vi "Main_direct.vi"() -> ()   [LabVIEW 2016]
doc: "The myRIO Project template acquires acceleration data from the onboard accelerometer and displays the changes of acceleration values in a waveform chart."
uses:
  <vilib>/FPGAPlugInAG/myRIO-1900/niLvFpga_Open_myRIO-1900.vi
  <vilib>/rvi/interface/common/dynamic/niFpgaDynamicAddResources.vi
  <vilib>/Utility/error.llb/Error Cluster From Error Code.vi
  <vilib>/rvi/errors/niLvFpgaAdjustHostInterfaceError.vi
  <vilib>/FPGAPlugInAG/Dynamic/niLvFpga_Close_Dynamic.vi
  <vilib>/rvi/interface/nirviOpenFPGA/nirviOpenFPGA.xnode
  FPGA Bitfiles/WS2811driver_FPGATarget_FPGAmain_HaK4FqHt+Z8.lvbitx
  <vilib>/rvi/interface/nirviReadWriteControl/nirviReadWriteControl.xnode
  <vilib>/rvi/interface/nirviCloseFPGA/nirviCloseFPGA.xnode
  NiFpgaLv.dll
  <vilib>/rvi/interface/Simulation/niFpgaSimulationCallBeginRW.vi
panel:
  in  "Numeric":u8=1
  out "Numeric Control 2":i32=155
  out "x^2":dbl=0.3694732795078815
  out "Boolean 3":bool=TRUE
  out "Boolean 2":bool
  out "Boolean":bool
  out "Numeric Control":i32=94
  out "appended array":bool[](array[boolean])=[FALSE, FALSE, FALSE, FALSE, FALSE, FALSE, FALSE, FALSE, FALSE, FALSE, FALSE, FALSE, FALSE, FALSE, FALSE, FALSE, FALSE, TRUE, FALSE, TRUE, TRUE, TRUE, TRUE, FALSE]
  in  "Count(mSec)":u32=25
  in  "H0":i32=20
  in  "L1":i32=52
  in  "L0":i32=80
  in  "H1":i32=48
  in  "Enum":enum16{"WS2812", "WS2811", "Debug"}(ring)
  in  "reset ticks)":u32=2000
  in  "number of leds":i32=100
  in  "Stop Button":bool
  out "error out":errorcluster={"status"=FALSE, "code"=-2220, "source"=""}
  # "Overview: The myRIO Project template acquires acceleration data from the onboard accelerometer and displays the changes of acceleration values in a waveform chart.\nInstructions:\n1. Check the myRIO target IP address in the project and make sure the target IP address is correct. \n2. Run this VI."
  # "g"
  # "b"
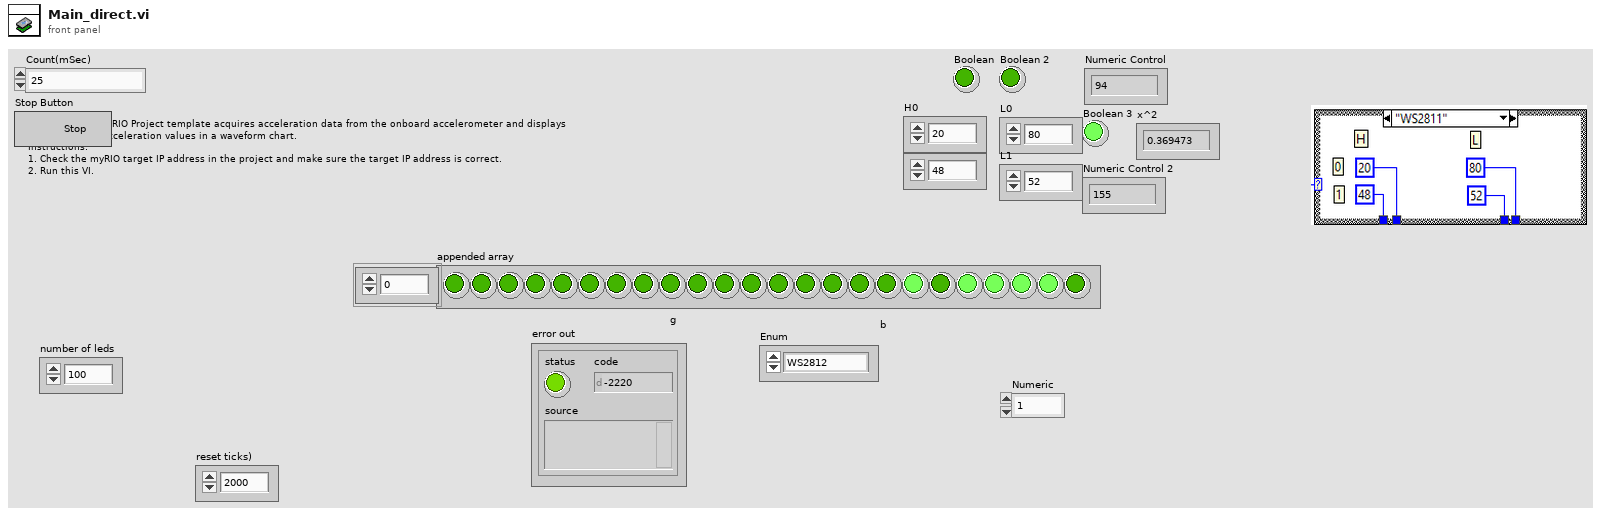
[diagram p1: front panel]
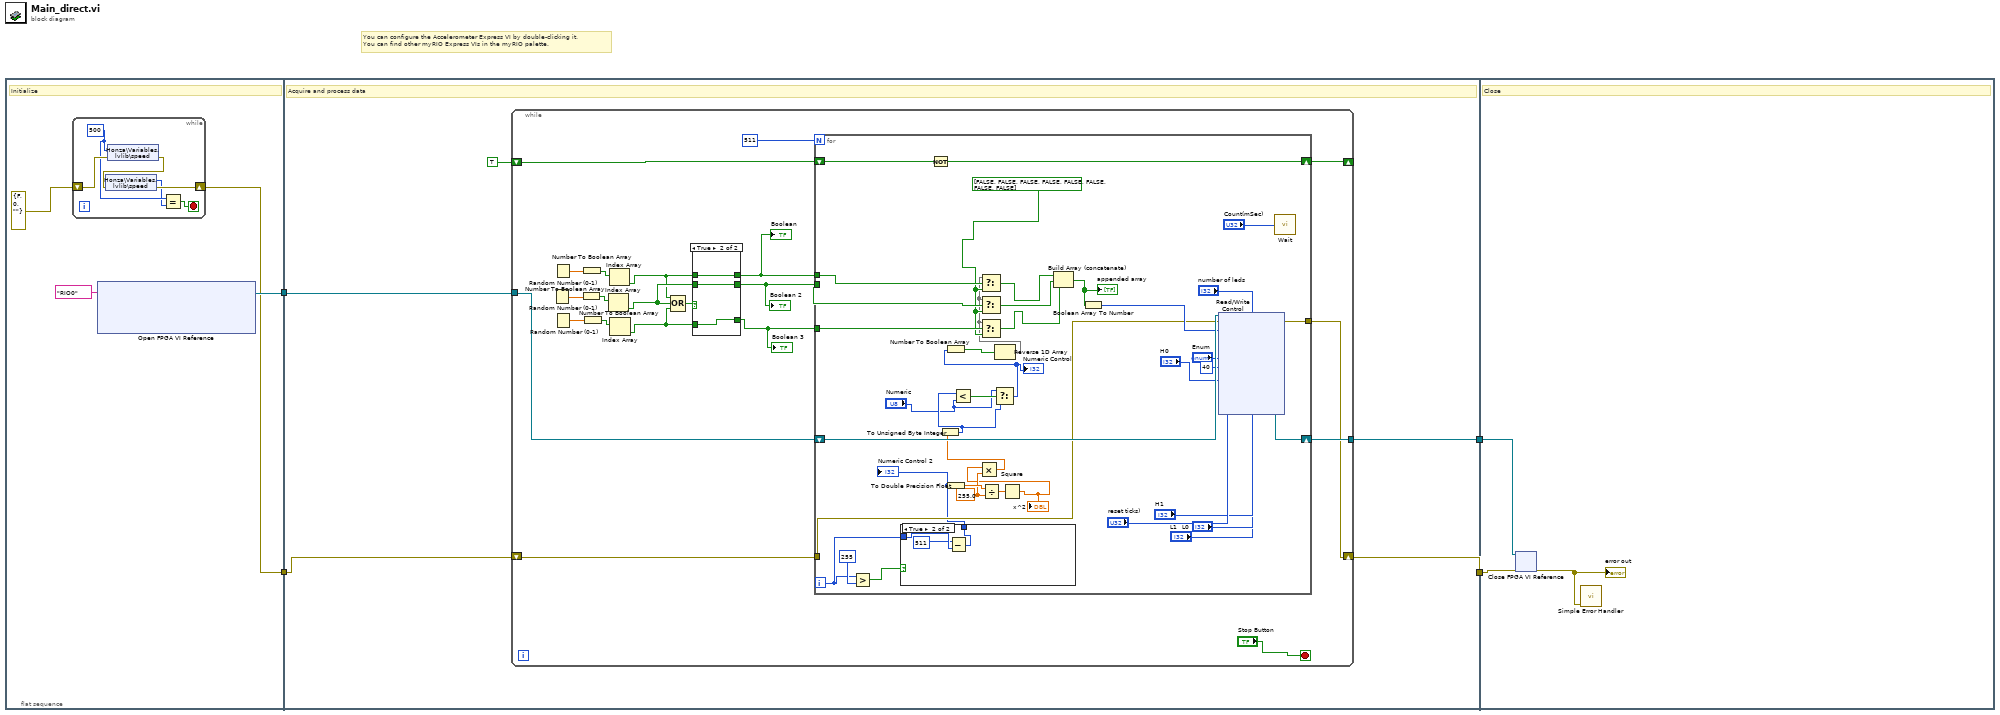
[diagram p0: block diagram]
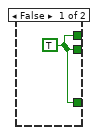
[diagram p2: hidden frame]
diagram:
  # "You can configure the Accelerometer Express VI by double-clicking it.\nYou can find other myRIO Express VIs in the myRIO palette."
  n1 = flat-sequence {
    tunnel: [w6] -> w4
    tunnel: [w8] -> w2
    tunnel: w4 -> [w18]
    tunnel: [w19] -> w3
    tunnel: w2 -> [w17]
    tunnel: [w16] -> w1
    tunnel: w3 -> [w90]
    tunnel: w1 -> [w88]
    frame #0 {
      # "Initialize"
      n2 = while {
        shift-right: [w14] -> w6
        shift-left: errorcluster {"status"=FALSE, "code"=0, "source"=""} ("error in (no error)") -> [w13]
        stop <- w11 stop-if-true
        w10 = 500 ("speed")
        n3 = shared-variable "Honza\\Variables.lvlib\\speed"(w10, error in=w13) -> (error out=w12:errorcluster)
        n4 = shared-variable "Honza\\Variables.lvlib\\speed"(error in=w12) -> (w9:i32, error out=w14:errorcluster)
        n5 = Equal?(x=w10, y=w9) -> (x = y?=w11:bool)
      }
      n6 = xnode "Open FPGA VI Reference"("resource name"=tag "RIO0") -> ("FPGA VI Reference Out"=w8:refnum<k20>)  [unwired: 1 in, 1 out]
    }
    frame #1 {
      # "Acquire and process data"
      n7 = while {
        shift-right: [w34] -> w19
        shift-left: w18 -> [w35]
        tunnel: w17 -> [w40]
        tunnel: [w38] -> w16
        shift-right: [w37] -> _
        shift-left: TRUE -> [w36]
        stop <- "Stop Button" stop-if-true
        n8 = Random Number (0-1)() -> (number: 0 to 1=w29:dbl)
        n9 = Random Number (0-1)() -> (number: 0 to 1=w32:dbl)
        n10 = Random Number (0-1)() -> (number: 0 to 1=w28:dbl)
        n11 = Number To Boolean Array(number=w29) -> (Boolean array=w30:bool[])
        n12 = Number To Boolean Array(number=w32) -> (Boolean array=w31:bool[])
        n13 = Number To Boolean Array(number=w28) -> (Boolean array=w27:bool[])
        n14 = Index Array(array=w30) -> (element=w24:bool)  [unwired: 1 in]
        n15 = Index Array(array=w31) -> (element=w23:bool)  [unwired: 1 in]
        n16 = Index Array(array=w27) -> (element=w25:bool)  [unwired: 1 in]
        n17 = Compound Arithmetic op=OR(w23, w24, w25) -> (w26:bool)
        n18 = case shown="True" w26 {
          tunnel: w23 -> [_ w44]
          tunnel: w24 -> [_ w43]
          tunnel: w25 -> [_ w42]
          tunnel: [w41 w44] -> w22
          tunnel: [w41 w43] -> w21
          tunnel: [w41 w42] -> w20
          frame False {
            w41 = TRUE
          }
          frame True {
          }
        }
        "Boolean" <- w22
        "Boolean 2" <- w21
        "Boolean 3" <- w20
        n19 = for {
          N: 511 -> [_]
          shift-right: [w82] -> w38
          shift-left: w40 -> [w83]
          shift-right: [w78] -> w37
          shift-left: w36 -> [w71]
          tunnel: w35 -> [w70]
          tunnel: [w69] -> w34
          tunnel: w22 -> [w62]
          tunnel: w20 -> [w61]
          tunnel: w21 -> [w60]
          i -> [w55]
          w51 = 255.0 ("y")
          w58 = bool[] [FALSE, FALSE, FALSE, FALSE, FALSE, FALSE, FALSE, FALSE]
          n20 = Greater?(x=w55, y=255 ("x")) -> (0:w67:bool)
          n21 = case shown="True" w67 {
            tunnel: w55 -> [w84 w86]
            tunnel: [w84 w87] -> w54
            frame False {
            }
            frame True {
              n22 = Subtract(x=511 ("y"), y=w86) -> (x-y=w87:i32)
            }
          }
          "Numeric Control 2" <- w54
          n23 = Not(x=w71) -> (.not. x?=w78:bool)
          n24 = To Double Precision Float(number=w54) -> (double precision float=w53:dbl)
          n25 = Divide(x=w53, y=w51) -> (x/y=w52:dbl)
          n26 = Square(x=w52) -> (x^2=w50:dbl)
          "x^2" <- w50
          n27 = Multiply(x=w50, y=w51) -> (x*y=w49:dbl)
          n28 = To Unsigned Byte Integer(number=w49) -> (unsigned 8bit integer=w46:u8)
          n29 = Less?(x=w46, y="Numeric") -> (x < y?=w48:bool)
          n30 = Select(t="Numeric", s=w48, f=w46) -> (s? t:f=w47:u8)
          "Numeric Control" <- w47
          n31 = Number To Boolean Array(number=w47) -> (Boolean array=w59:bool[])
          n32 = Reverse 1D Array(array=w59) -> (reversed array=w57:bool[])
          n33 = Select(t=w57, s=w62, f=w58) -> (s? t:f=w66:bool[])
          n34 = Select(t=w57, s=w60, f=w58) -> (s? t:f=w65:bool[])
          n35 = Select(t=w57, s=w61, f=w58) -> (s? t:f=w64:bool[])
          n36 = Build Array (concatenate)(w66, w65, w64) -> (w63:bool[])
          "appended array" <- w63
          n37 = Boolean Array To Number(Boolean array=w63) -> (number=w81:u32)
          n38 = xnode "Read/Write Control"("FPGA VI Reference In"=w83, "error in"=w70, "color"=w81, "number of leds"="number of leds", "reset ticks)"="reset ticks)", "Enum"="Enum", "looptime"=u32 40, "H0"="H0", "H1"="H1", "L0"="L0", "L1"="L1") -> ("FPGA VI Reference Out"=w82:refnum<k20>, "error out"=w69:errorcluster)
          n39 = call "Wait"("Count(mSec)"="Count(mSec)") -> ()  [unwired: 1 out]
        }
      }
    }
    frame #2 {
      # "Close"
      n40 = xnode "Close FPGA VI Reference"("FPGA VI Reference In"=w88, "error in"=w90) -> ("error out"=w89:errorcluster)
      "error out" <- w89
      n41 = call <vilib>:"Simple Error Handler.vi"("error in (no error)"=w89) -> ()  [unwired: 4 in, 5 out]
    }
  }
